vi "get_nominal_soft_limit.vi"(3 "error in (no error)":errorcluster caption="错误输入（无错误）", 6 "OneMotion 输入":refnum<class "OneMotion.lvclass">) -> (0 "error out":errorcluster caption="错误输出", 1 "nominal soft limit (considering the backlash compensation)":cluster{"min":dbl, "max":dbl}, 2 "OneMotion 输出":refnum<class "OneMotion.lvclass">)   [LabVIEW 2014, in "OneMotion.lvclass"]
uses:
  OneMotion.lvclass
  OneMotion.lvclass/OneMotion.ctl
panel:
  # "This has a bug:\nwhat if the current pos is already \nout of the nominal soft limit?"
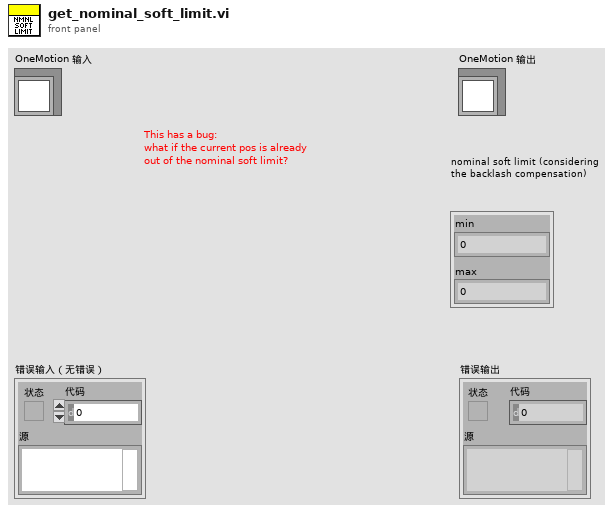
[diagram p1: front panel]
types:
  T1 = typedef "OneMotion.lvclass/backlash option.ctl" = enum16{"no backlash compensation", "compensation: from - to +", "compensation: from + to -"}
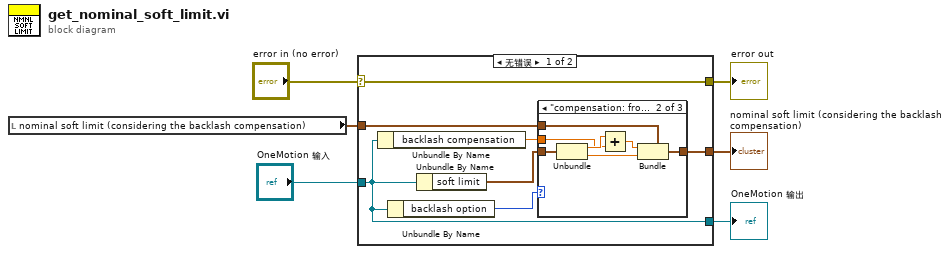
[diagram p0: block diagram]
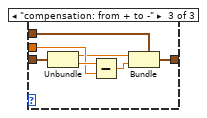
[diagram p3: hidden frame]
diagram:
  n1 = local read "nominal soft limit (considering the backlash compensation)"() -> (w1:cluster{"min":dbl, "max":dbl})
  n2 = case shown="无错误" "error in (no error)" {
    selector: "error in (no error)" -> [w13 w31]
    tunnel: [w13 w31] -> w5
    tunnel: [w11 w30] -> w3
    tunnel: "OneMotion 输入" -> [w11 w30]
    tunnel: [w8 w29] -> w2
    tunnel: w1 -> [w7 w29]
    frame No Error {
      n3 = Unbundle By Name(w11) -> ("backlash compensation"=w10:dbl)
      n4 = Unbundle By Name(w11) -> ("backlash option"=w12:T1)
      n5 = Unbundle By Name(w11) -> ("soft limit"=w9:cluster{"min":dbl, "max":dbl})
      n6 = case shown="\"compensation: from - to +\"" w12 {
        tunnel: w10 -> [_ w19 w26]
        tunnel: w9 -> [w14 w21 w28]
        tunnel: [w14 w16 w23] -> w8
        tunnel: w7 -> [_ w15 w22]
        frame "no backlash compensation", Default {
        }
        frame "compensation: from - to +" {
          n7 = Unbundle(w21) -> ("min"=w20:dbl, "max"=w17:dbl)
          n8 = Add(x=w20, y=w19) -> (x+y=w18:dbl)
          n9 = Bundle(cluster=w15, "min"=w18, "max"=w17) -> (w16:cluster{"min":dbl, "max":dbl})
        }
        frame "compensation: from + to -" {
          n10 = Unbundle(w28) -> ("min"=w25:dbl, "max"=w27:dbl)
          n11 = Subtract(x=w27, y=w26) -> (x-y=w24:dbl)
          n12 = Bundle(cluster=w22, "min"=w25, "max"=w24) -> (w23:cluster{"min":dbl, "max":dbl})
        }
      }
    }
    frame Error {
    }
  }
  "error out" <- w5
  "OneMotion 输出" <- w3
  "nominal soft limit (considering the backlash compensation)" <- w2
